vi "Determine Optimal Setpoints - Alternate Method.vi"(0 "Front Left":dbl, 2 "Front Right":dbl, 4 "Rear Left":dbl, 6 "Rear Right":dbl) -> (20 "Front Left Out":dbl, 21 "Front Right Out":dbl, 22 "Rear Left Out":dbl, 23 "Rear Right Out":dbl, 24 "Inv. Front Left Drive?":bool, 25 "Inv. Front Right Drive?":bool, 26 "Inv. Rear Left Drive?":bool, 27 "Inv. Rear Right Drive?":bool)   [LabVIEW 2011]
uses:
  Globals/Potentiometers.vi
panel:
  # "These are taken in as angles and output as absolute pot voltage."
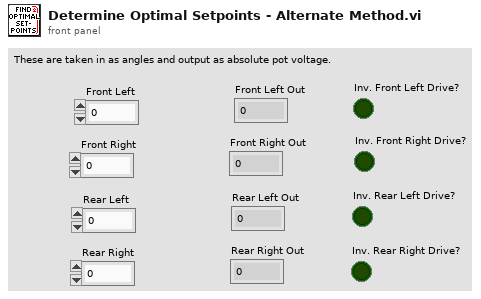
[diagram p1: front panel]
types:
  T1 = typedef "WPI_AnalogChannelDevRef.ctl" = cluster{"DevStatus":errorcluster, "Analog Module":T2, "Analog Channel":T3}
  T2 = typedef "FPGA_TypedefAnalogModule.ctl" = enum16{"Analog Module 1", "Analog Module 2"}
  T3 = typedef "FPGA_AIChannel.ctl" = enum8{"AI 1", "AI 2", "AI 3", "AI 4", "AI 5", "AI 6", "AI 7", "AI 8", "Invalid"}
  T4 = cluster{"Front Left":T1, "Front Right":T1, "Rear Left":T1, "Rear Right":T1, "Actuator":T1}
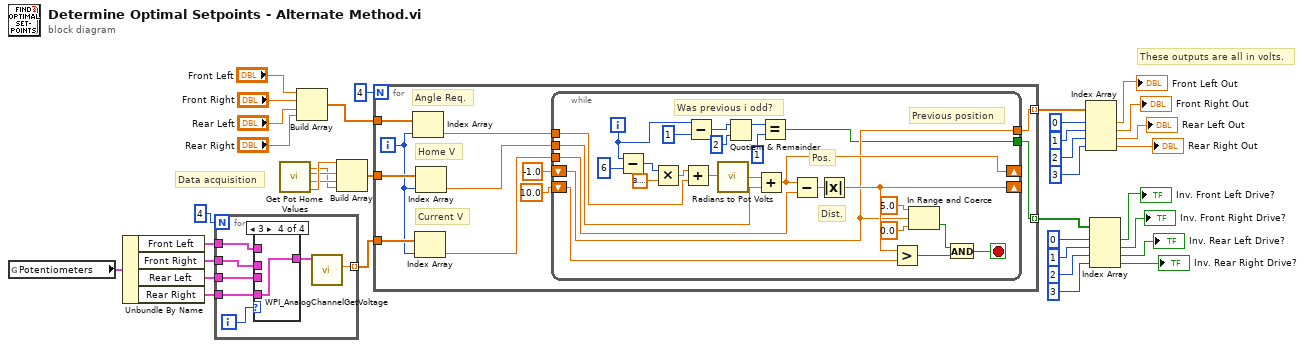
[diagram p0: block diagram]
diagram:
  # "Data acquisition"
  # "These outputs are all in volts."
  n1 = global read "Potentiometers.vi" "Potentiometers"() -> (w28:T4)
  n2 = Unbundle By Name(w28) -> ("Front Left"=w26:T1, "Front Right"=w25:T1, "Rear Left"=w24:T1, "Rear Right"=w23:T1)
  n3 = for {
    N: 4 -> [_]
    tunnel: w26 -> [w42]
    tunnel: w25 -> [w41]
    tunnel: w24 -> [w40]
    tunnel: w23 -> [w39]
    tunnel: [w37] -> w19 mode=indexing
    i -> [w43]
    n4 = case shown="3" w43 {
      tunnel: w42 -> [w44 _ _ _]
      tunnel: w41 -> [_ w45 _ _]
      tunnel: w40 -> [_ _ w46 _]
      tunnel: w39 -> [_ _ _ w47]
      tunnel: [w44 w45 w46 w47] -> w38
      frame 0, Default {
      }
      frame 1 {
      }
      frame 2 {
      }
      frame 3 {
      }
    }
    n5 = call <vilib>:"WPI_AnalogChannelGetVoltage.vi"("AIDeviceRef"=w38) -> ("Voltage"=w37:dbl)  [unwired: 8 in, 2 out]
  }
  n6 = call "Get Pot Home Values.vi"() -> ("Front Left"=w32:dbl, "Rear Left"=w30:dbl, "Front Right"=w31:dbl, "Rear Right"=w29:dbl)  [unwired: 8 in]
  n7 = Build Array("Front Left", "Front Right", "Rear Left", "Rear Right") -> (w21:dbl[])
  n8 = Build Array(w32, w31, w30, w29) -> (w20:dbl[])
  n9 = for {
    N: 4 -> [_]
    tunnel: w21 -> [w58]
    tunnel: w20 -> [w57]
    tunnel: w19 -> [w56]
    tunnel: [w48] -> w2 mode=indexing
    tunnel: [w49] -> w1 mode=indexing
    i -> [w55]
    # "Current V"
    # "Home V"
    # "Angle Req."
    n10 = Index Array(array=w58, index=w55) -> (element=w54:dbl)
    n11 = Index Array(array=w56, index=w55) -> (element=w52:dbl)
    n12 = Index Array(array=w57, index=w55) -> (element=w53:dbl)
    n13 = while {
      tunnel: w54 -> [w83]
      tunnel: w53 -> [w84]
      shift-right: [w71] -> _
      shift-left: -1.0 -> [w67]
      tunnel: w52 -> [w82]
      shift-right: [w74] -> _
      shift-left: 10.0 -> [w75]
      tunnel: [w67] -> w49
      tunnel: [w59] -> w48
      i -> [w60]
      stop <- w70 stop-if-true
      # "Previous position"
      # "Was previous i odd?"
      # "Dist."
      # "Pos."
      n14 = Subtract(x=w60, y=6) -> (x-y=w77:i32)
      n15 = Multiply(x=w77, y=3.141592653589793) -> (x*y=w80:dbl)
      n16 = Add(x=w80, y=w83) -> (x+y=w79:dbl)
      n17 = Subtract(x=w60, y=1) -> (x-y=w64:i32)
      n18 = call "Radians to Pot Volts.vi"("Angle In"=w79) -> ("Pot Delta Out"=w78:dbl)
      n19 = Quotient & Remainder(x=w64, y=2) -> (x-y*floor(x/y)=w62:i32)  [unwired: 1 out]
      n20 = Add(x=w78, y=w84) -> (x+y=w71:dbl)
      n21 = Equal?(x=w62, y=1) -> (x = y?=w59:bool)
      n22 = Subtract(x=w71, y=w82) -> (x-y=w81:dbl)
      n23 = Absolute Value(x=w81) -> (abs(x)=w74:dbl)
      n24 = Greater?(x=w74, y=w75) -> (0:w69:bool)
      n25 = In Range and Coerce(upper limit=5.0, x=w67, lower limit=0.0) -> (In Range?=w68:bool)  [unwired: 1 out]
      n26 = And(x=w68, y=w69) -> (x .and. y?=w70:bool)
    }
  }
  n27 = Index Array(array=w1, index #1=0 ("index"), index #2=1 ("index"), index #3=2 ("index"), index #4=3 ("index")) -> (element #1=→"Front Left Out":dbl, element #2=→"Front Right Out":dbl, element #3=→"Rear Left Out":dbl, element #4=→"Rear Right Out":dbl)
  n28 = Index Array(array=w2, index #1=0 ("index"), index #2=1 ("index"), index #3=2 ("index"), index #4=3 ("index")) -> (element #1=→"Inv. Front Left Drive?":bool, element #2=→"Inv. Front Right Drive?":bool, element #3=→"Inv. Rear Left Drive?":bool, element #4=→"Inv. Rear Right Drive?":bool)
